vi "Manual Triggered B-Scan Interrupted.vi"() -> ()   [LabVIEW 2012]
uses:
  LabVIEW/user.lib/SpectralRadar.llb/Processing Flag Selection.ctl
  LabVIEW/user.lib/SpectralRadar.llb/Normal Direction Selection.ctl
  LabVIEW/user.lib/SpectralRadar.llb/display Data 2D.vi
  LabVIEW/user.lib/SpectralRadar.llb/set Offset Corrected Spectrum Output.vi
  LabVIEW/user.lib/SpectralRadar.llb/OCT Device.lvclass
  LabVIEW/user.lib/SpectralRadar.llb/Processing.lvclass
  LabVIEW/user.lib/SpectralRadar.llb/Raw Data.lvclass
  LabVIEW/user.lib/SpectralRadar.llb/Data.lvclass
  LabVIEW/user.lib/SpectralRadar.llb/Scan Pattern.lvclass
panel:
  out "Current Chunk":i32
  in  "Chunks":i32=10
  in  "stop":bool
  out "Intensity Graph":dbl[][](graph)
  in  "Chunk Size":i32=256
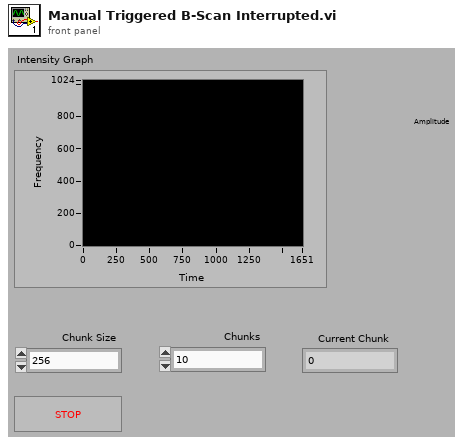
[diagram p1: front panel]
types:
  T1 = typedef "Processing.lvclass/Processing Flag Selection.ctl" = enum16{"Use Offset Errors", "Remove DC Spectrum", "Remove Advanced DC Spectrum", "Use Apodization", "Use Scan For Apodization", "Filter Undersampled Signals", "Use Dispersion Compensation", "Use Dechirp", "Use Extended Adjust", "Full Range Output", "Filter DC", "Autocorrelation Compensation", "DEFR", "Only Windowing", "Remove Fixed Pattern"}
  T2 = enum16{"Asynchronous Continuous", "Asynchronous Finite", "Synchronous"}
  T3 = typedef "Data.lvclass/Normal Direction Selection.ctl" = enum16{"Direction 1", "Direction 2", "Direction 3"}
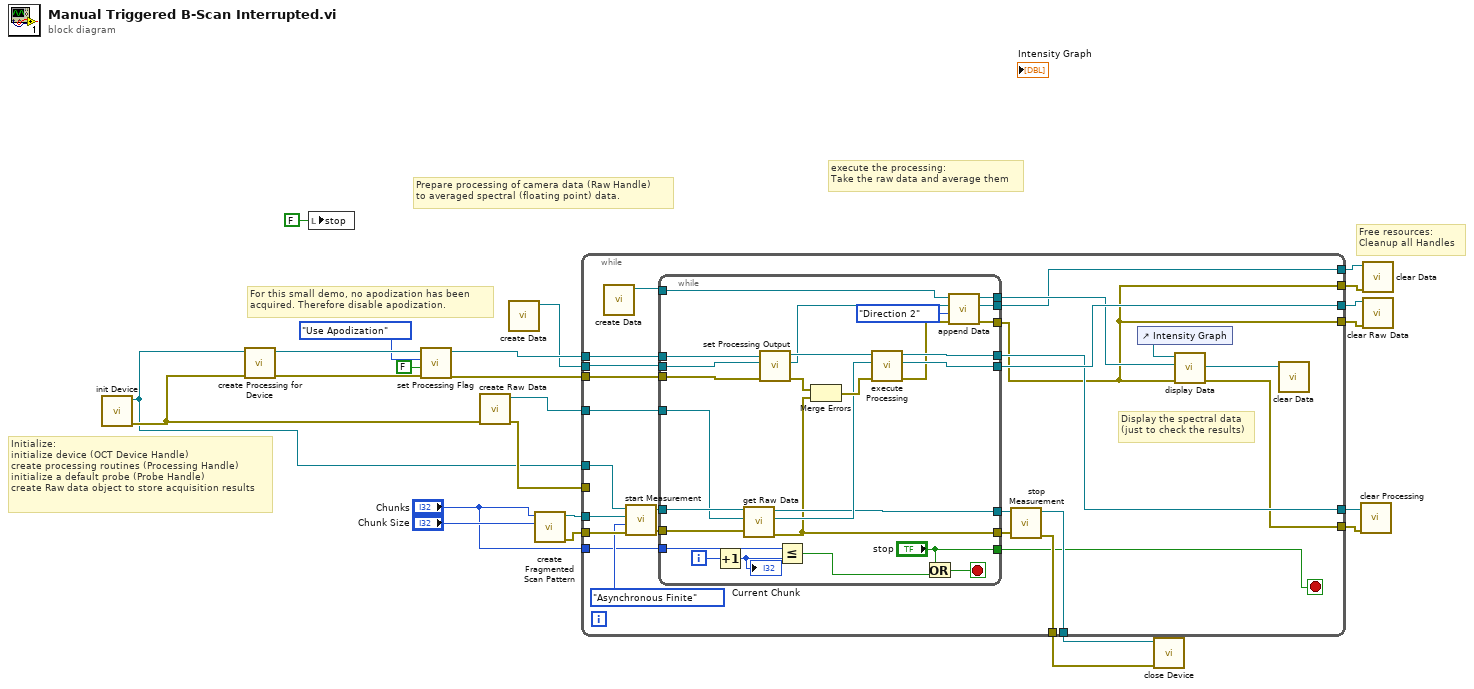
[diagram p0: block diagram]
diagram:
  # "execute the processing:\nTake the raw data and average them"
  # "For this small demo, no apodization has been \nacquired. Therefore disable apodization."
  # "Free resources:\nCleanup all Handles"
  # "Prepare processing of camera data (Raw Handle)\nto averaged spectral (floating point) data."
  # "Initialize:\ninitialize device (OCT Device Handle)\ncreate processing routines (Processing Handle)\ninitialize a default probe (Probe Handle)\ncreate Raw data object to store acquisition results"
  n1 = call "init Device.vi"() -> ("error out"=w24:errorcluster, "OCTDevice"=w12:refnum<class "OCT Device.lvclass">)  [unwired: 6 in]
  n2 = call "create Processing for Device.vi"("error in (no error)"=w24, "OCTDevice"=w12) -> ("error out"=w15:errorcluster, "Processing"=w19:refnum<class "Processing.lvclass">)  [unwired: 3 in, 1 out]
  n3 = local write "stop"(FALSE ("stop")) -> ()
  n4 = call "set Processing Flag.vi"("error in (no error)"=w15, "Flag"=FALSE, "Processing Flag Selection"=Processing_Flag_Selection."Use Apodization", "Processing"=w19) -> ("error out"=w16:errorcluster, "Processing"=w18:refnum<class "Processing.lvclass">)  [unwired: 2 in]
  n5 = call "create Raw Data.vi"("error in (no error)"=w24) -> ("error out"=w13:errorcluster, "Raw Data"=w23:refnum<class "Raw Data.lvclass">)  [unwired: 5 in]
  n6 = call "create Data.vi"() -> ("Data"=w3:refnum<class "Data.lvclass">)  [unwired: 6 in, 1 out]
  n7 = call "create Fragmented Scan Pattern.vi"("Chunk Size"="Chunk Size", "Number of Chunks"="Chunks") -> ("error out"=w10:errorcluster, "Scan Pattern"=w11:refnum<class "Scan Pattern.lvclass">)  [unwired: 4 in]
  n8 = while {
    tunnel: w23 -> [w39]
    tunnel: w3 -> [w49]
    tunnel: w12 -> [w42]
    tunnel: [w48] -> w22
    tunnel: [w47] -> w21
    tunnel: [w28] -> w20
    tunnel: w18 -> [w46]
    tunnel: w16 -> [w45]
    tunnel: w13 -> [_]
    tunnel: w11 -> [w43]
    tunnel: w10 -> [w41]
    tunnel: [w36] -> w8
    tunnel: "Chunks" -> [w33]
    tunnel: [w32] -> w6
    tunnel: [w30] -> w5
    tunnel: [w29] -> w2
    tunnel: [w28] -> w1
    stop <- w27 stop-if-true
    # "Display the spectral data\n(just to check the results)"
    n9 = call "create Data.vi"() -> ("Data"=w26:refnum<class "Data.lvclass">)  [unwired: 6 in, 1 out]
    n10 = call "start Measurement.vi"("error in (no error)"=w41, "Acquisition Type"=T2."Asynchronous Finite", "Scan Pattern"=w43, "OCTDevice"=w42) -> ("error out"=w38:errorcluster, "OCTDevice"=w40:refnum<class "OCT Device.lvclass">)  [unwired: 1 in, 1 out]
    n11 = while {
      tunnel: w49 -> [w76]
      tunnel: [w74] -> w48
      tunnel: [w71] -> w47
      tunnel: w46 -> [w70]
      tunnel: w45 -> [w69]
      tunnel: w40 -> [w68]
      tunnel: w39 -> [w67]
      tunnel: w38 -> [w66]
      tunnel: [w64] -> w37
      tunnel: [w63] -> w35
      tunnel: w33 -> [w62]
      tunnel: w26 -> [w60]
      tunnel: [w57] -> w31
      tunnel: [w56] -> w29
      tunnel: [w55] -> w28
      tunnel: ["stop"] -> w27
      i -> [w61]
      stop <- w53 stop-if-true
      n12 = Increment(x=w61) -> (x+1=w51:i32)
      "Current Chunk" <- w51
      n13 = call "get Raw Data.vi"("error in (no error)"=w66, "RawData in"=w67, "OCTDevice in"=w68) -> ("error out"=w63:errorcluster, "RawData out"=w65:refnum<class "Raw Data.lvclass">, "OCTDevice out"=w64:refnum<class "OCT Device.lvclass">)  [unwired: 2 in]
      n14 = call-poly "set Processing Output.vi"("error in (no error)"=w69, "Data"=w76, "Processing"=w70) -> ("error out"=w73:errorcluster, "Data"=w59:refnum<class "Data.lvclass">, "Processing"=w75:refnum<class "Processing.lvclass">)  [unwired: 2 in]
      n15 = Less Or Equal?(x=w62, y=w51) -> (x <= y?=w52:bool)
      n16 = Merge Errors(w73, w63) -> (w72:errorcluster)
      n17 = call "execute Processing.vi"("error in (no error)"=w72, "Raw Data"=w65, "Processing"=w75) -> ("error out"=w58:errorcluster, "Raw Data"=w74:refnum<class "Raw Data.lvclass">, "Processing"=w71:refnum<class "Processing.lvclass">)  [unwired: 2 in]
      n18 = Or(x="stop", y=w52) -> (x .or. y?=w53:bool)
      n19 = call "append Data.vi"("error in (no error)"=w58, "Normal Direction"=Normal_Direction_Selection."Direction 2", "Data to append in"=w59, "Data in"=w60) -> ("error out"=w55:errorcluster, "Data to append out"=w56:refnum<class "Data.lvclass">, "Data out"=w57:refnum<class "Data.lvclass">)  [unwired: 1 in]
    }
    n20 = call "stop Measurement.vi"("error in (no error)"=w35, "OCTDevice"=w37) -> ("error out"=w32:errorcluster, "OCTDevice"=w36:refnum<class "OCT Device.lvclass">)  [unwired: 4 in]
    n21 = control-ref of="Intensity Graph"() -> (w44:refnum<vi>)
    n22 = call-poly "display Data.vi"("error in (no error)"=w28, "Data in"=w31, "IntGraph Refnum"=w44) -> ("error out"=w30:errorcluster, "Data out"=w25:refnum<class "Data.lvclass">)  [unwired: 2 in, 1 out]
    n23 = call "clear Data.vi"("Data"=w25) -> ()  [unwired: 6 in, 1 out]
  }
  n24 = call "close Device.vi"("error in (no error)"=w6, "OCTDevice"=w8) -> ()  [unwired: 5 in, 1 out]
  n25 = call "clear Processing.vi"("error in (no error)"=w5, "Processing"=w21) -> ()  [unwired: 5 in, 1 out]
  n26 = call "clear Data.vi"("error in (no error)"=w1, "Data"=w2) -> ()  [unwired: 5 in, 1 out]
  n27 = call "clear Raw Data.vi"("error in (no error)"=w20, "Raw Data"=w22) -> ()  [unwired: 5 in, 1 out]
